vi "PNG Picture Setup.vi"(6 "picture background":picture, 8 "error in (no error)":errorcluster, 11 "image data":T1) -> (0 "error out":errorcluster, 3 "picture":picture)   [LabVIEW 2021, in "Pop-Up.lvlib" / "PNG Parent.lvclass"]
doc: "read the information for the custom image \n\n<b>Code Developed By:</b> +\nDaniel Coons +\nhttps://github.com/danielcoons/tsc-pop-up"
uses:
  PNG Parent.lvclass
  <vilib>/picture/picture.llb/imagedata.ctl
  PNG Parent.lvclass/PNG Parent.ctl
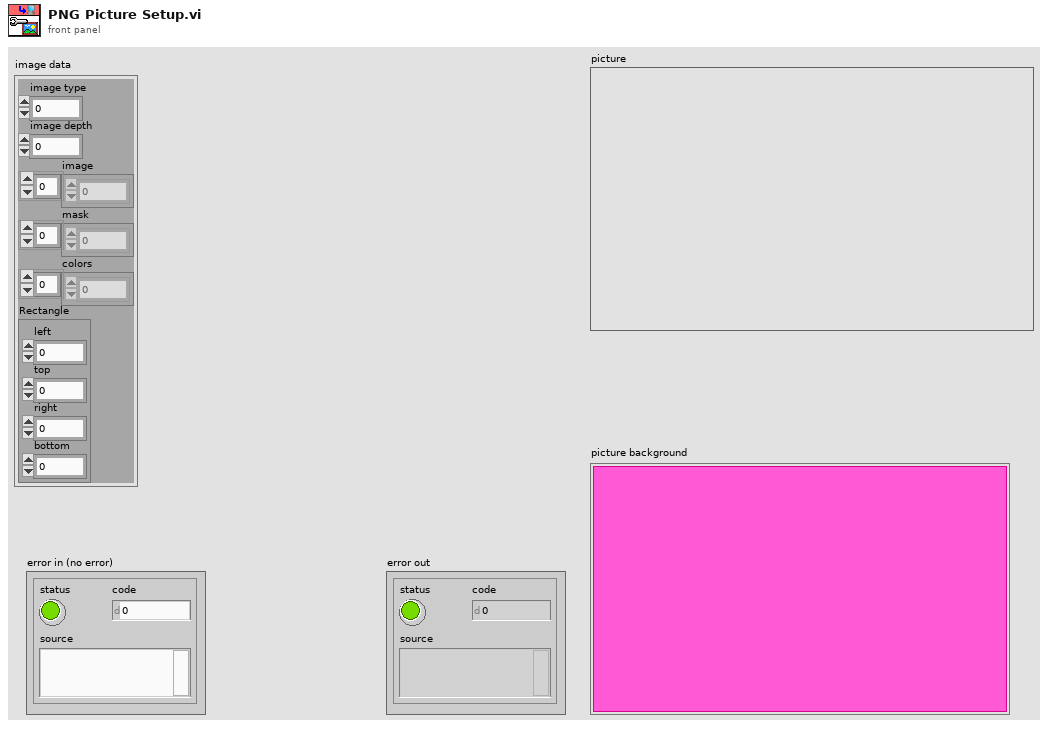
[diagram p1: front panel]
types:
  T1 = typedef "imagedata.ctl" = cluster{"image type":i32, "image depth":i32, "image":u8[], "mask":u8[], "colors":u32[], "Rectangle":cluster{"left":i16, "top":i16, "right":i16, "bottom":i16}}
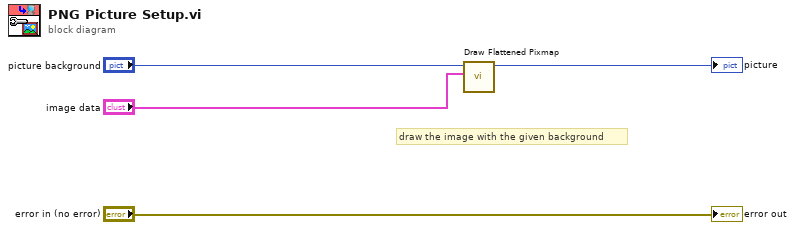
[diagram p0: block diagram]
diagram:
  # "draw the image with the given background"
  n1 = call <vilib>:"Draw Flattened Pixmap.vi"("image data"="image data", "picture"="picture background") -> ("new picture"=→"picture":picture)  [unwired: 7 in]
  "error out" <- "error in (no error)"
